vi "SystemController.ClassRefFGV.vi"(8 "error in (no error)":errorcluster, 10 "Set/Get":enum16{"Set", "Get"}(ring), 11 "SystemController":refnum<class "SystemController.lvclass">) -> (0 "error out":errorcluster, 3 "SystemController out":refnum<class "SystemController.lvclass">)   [LabVIEW 2017, in "SystemController.lvclass"]
doc: "---------------------------------------------------------------\nJKI State Machine Objects™\nhttp://jki.net/state-machine-objects/\nCopyright (C) 2005-2015, JKI <info@jki.net>\nALL RIGHTS RESERVEDJKI State Machine Objects (SMO) 1.0.0.5\nJKI - JKI\nCopyright (c) 2016, JKI"
uses:
  SystemController.lvclass
panel:
  # "For instructions on how to use the JKI State Machine Objects, examples and video tutorials, visit:\nhttp://jki.net/state-machine-objects/\n\nJKI State Machine Objects™\nhttp://jki.net/state-machine-objects/\nCopyright (C) 2005-2015, JKI <info@jki.net>\nALL RIGHTS RESERVED"
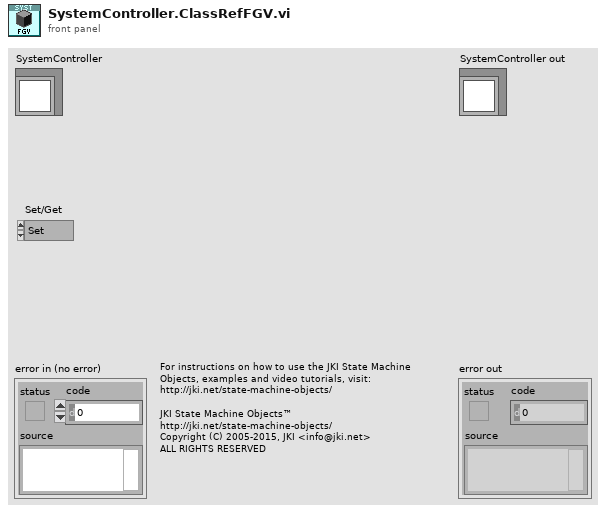
[diagram p1: front panel]
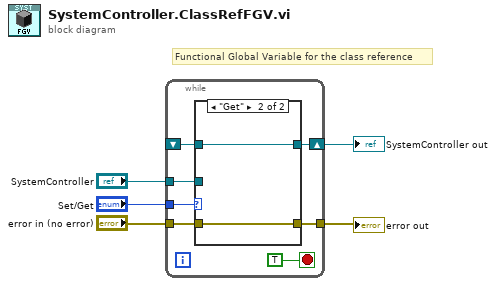
[diagram p0: block diagram]
diagram:
  # "Functional Global Variable for the class reference"
  n1 = while {
    tunnel: "Set/Get" -> [w11]
    shift-right: [w9] -> w4
    shift-left: _ -> [w10]
    tunnel: [w8] -> w3
    tunnel: "error in (no error)" -> [w7]
    tunnel: "SystemController" -> [w6]
    stop <- TRUE stop-if-true
    n2 = case shown="\"Get\"" w11 {
      tunnel: w10 -> [_ w16]
      tunnel: [w13 w16] -> w9
      tunnel: [w14 w15] -> w8
      tunnel: w7 -> [w14 w15]
      tunnel: w6 -> [w13 _]
      frame "Set", Default {
      }
      frame "Get" {
      }
    }
  }
  "error out" <- w3
  "SystemController out" <- w4
